vi "PositionControlCANTest.vi"() -> ()   [LabVIEW 2009, in "Test.lvlib"]
uses:
  Test.lvlib
  CAN/SubVIs/CAN Jaguar Control Mode.ctl
  OWNCAN.lvlib
  CAN.lvlib
panel:
  in  "stop 2":bool
  out "Output Right":dbl
  out "Output Left":dbl
  in  "D":dbl
  in  "I":dbl
  in  "P":dbl
  out "error out pid":errorcluster
  in  "Set PID":bool
  in  "Maximum Output Voltage":dbl=3.0
  out "error out hb":errorcluster
  out "error out close":errorcluster
  in  "Output Right":dbl
  in  "Output Left":dbl
  out "error out set out":errorcluster
  in  "stop":bool
  in  "Execute":bool
  in  "Control Mode":T1=enum."Position"
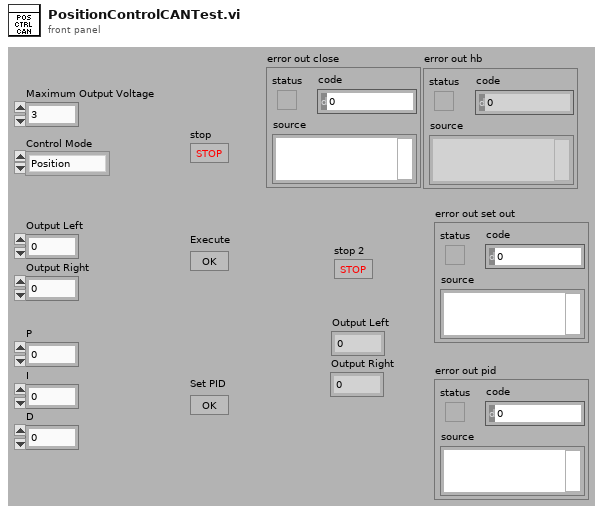
[diagram p1: front panel]
types:
  T1 = typedef "CAN.lvlib/CAN Jaguar Control Mode.ctl" = enum16{"Percent VBus", "Speed", "Position", "Current"}
  T2 = typedef "OWNCAN.lvlib/CAN Jaguars Ref.ctl" = cluster{"CAN Jaguar Ref Left":T3, "CAN Jaguar Ref Right":T3}
  T3 = typedef "CAN.lvlib/CAN Jaguar Ref.ctl" = cluster{"Device Number":u8, "Control Mode":T1, "Inverted":bool, "Semaphore":T4, "Max Vout":dbl, "DevStatus":errorcluster}
  T4 = typedef "Semaphore RefNum" = refnum<k1>
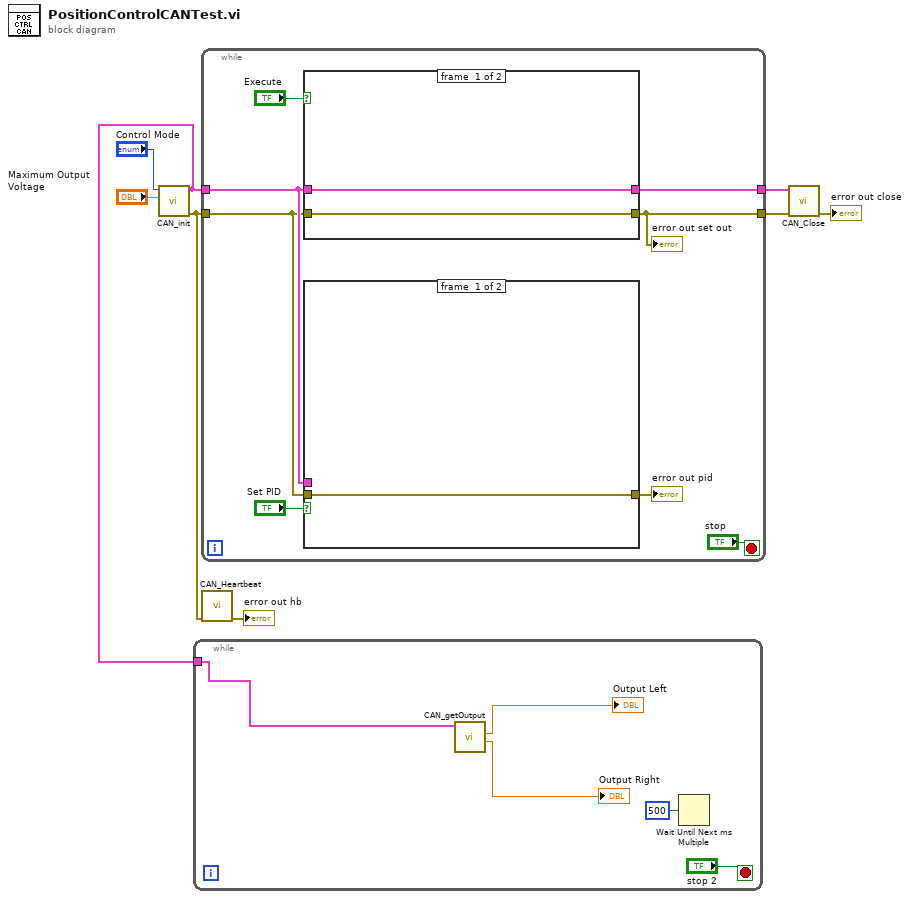
[diagram p0: block diagram]
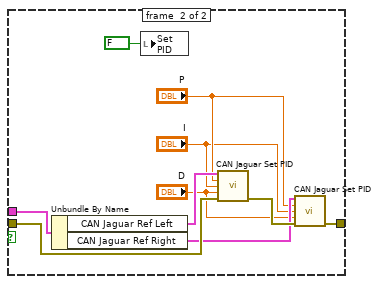
[diagram p2: hidden frame]
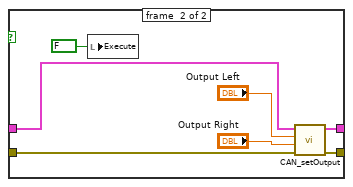
[diagram p3: hidden frame]
diagram:
  n1 = call "CAN_init.vi"("Maximum Output Voltage"="Maximum Output Voltage", "Control Mode"="Control Mode") -> ("error out"=w7:errorcluster, "CAN Jaguars Ref"=w1:T2)  [unwired: 6 in]
  n2 = while {
    tunnel: w1 -> [w11]
    stop <- "stop 2" stop-if-true
    n3 = call "CAN_getOutput.vi"("CAN Jaguars Ref"=w11) -> ("Right output"=→"Output Right":dbl, "Left output"=→"Output Left":dbl)  [unwired: 7 in, 2 out]
    n4 = Wait Until Next ms Multiple(millisecond multiple=u32 500) -> ()  [unwired: 1 out]
  }
  n5 = while {
    tunnel: w7 -> [w14]
    tunnel: [w19] -> w6
    tunnel: w1 -> [w15]
    tunnel: [w18] -> w5
    stop <- "stop" stop-if-true
    n6 = case shown="False" "Execute" {
      tunnel: w14 -> [w34 w40]
      tunnel: [w34 w39] -> w19
      tunnel: w15 -> [w33 w36]
      tunnel: [w33 w35] -> w18
      frame #0 {
      }
      frame #1 {
        n7 = local write "Execute"(FALSE ("OK Button")) -> ()
        n8 = call "CAN_setOutput.vi"("error in (no error)"=w40, "Output Right"="Output Right", "Output Left"="Output Left", "CAN Jaguars Ref"=w36) -> ("error out"=w39:errorcluster, "CAN Jaguars Ref out"=w35:T2)  [unwired: 6 in]
      }
    }
    "error out set out" <- w19
    n9 = case shown="False" "Set PID" {
      tunnel: w14 -> [w22 w29]
      tunnel: [w22 w27] -> w16
      tunnel: w15 -> [_ w31]
      frame #0 {
      }
      frame #1 {
        n10 = Unbundle By Name(w31) -> ("CAN Jaguar Ref Left"=w30:T3, "CAN Jaguar Ref Right"=w26:T3)
        n11 = local write "Set PID"(FALSE ("OK Button")) -> ()
        n12 = call "CAN Jaguar Set PID.vi"("CAN Jaguar Ref"=w30, "P"="P", "I"="I", "D"="D", "error in (no error)"=w29) -> ("error out"=w28:errorcluster)  [unwired: 9 in, 1 out]
        n13 = call "CAN Jaguar Set PID.vi"("CAN Jaguar Ref"=w26, "P"="P", "I"="I", "D"="D", "error in (no error)"=w28) -> ("error out"=w27:errorcluster)  [unwired: 9 in, 1 out]
      }
    }
    "error out pid" <- w16
  }
  n14 = call "CAN_Heartbeat.vi"("error in"=w7) -> ("error out"=→"error out hb":errorcluster)  [unwired: 10 in]
  n15 = call "CAN_Close.vi"("error in"=w6, "CAN Jaguars Ref"=w5) -> ("error out"=→"error out close":errorcluster)  [unwired: 9 in]
